vi "FPGA_v1.vi"() -> ()   [LabVIEW 2017]
panel:
  out "T":sgl
  in  "h":sgl format="%#_13g"
  out "norm(V)":sgl
  out "AoA_Yaw":sgl
  out "AoA_Pitch":sgl
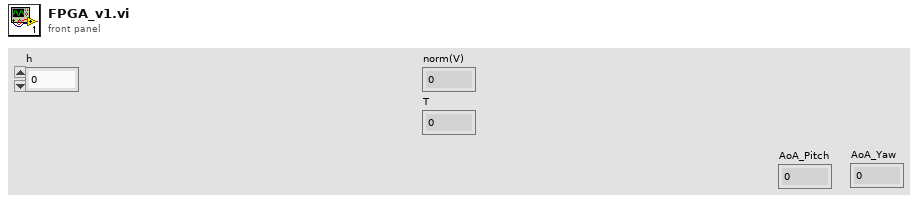
[diagram p1: front panel]
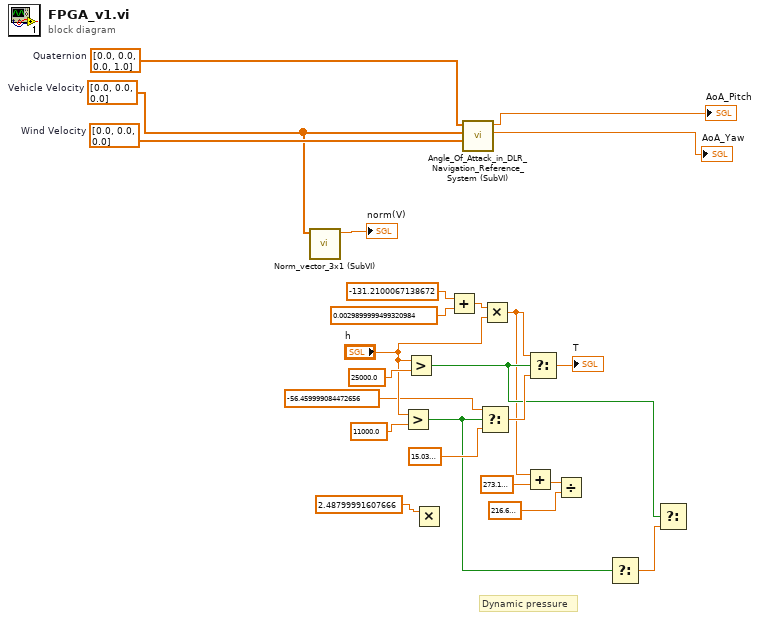
[diagram p0: block diagram]
diagram:
  w23 = sgl[] [0.0, 0.0, 0.0]  # Wind Velocity
  w20 = sgl[] [0.0, 0.0, 0.0]  # Vehicle Velocity
  w24 = sgl[] [0.0, 0.0, 0.0, 1.0]  # Quaternion
  # "Dynamic pressure"
  n1 = call "Norm_vector_3x1 (SubVI).vi"("Vector"=w20) -> ("Norm"=→"norm(V)":sgl)  [unwired: 10 in]
  n2 = Greater?(x="h", y=sgl 11000.0) -> (0:w6:bool)
  n3 = Greater?(x="h", y=sgl 25000.0) -> (0:w7:bool)
  n4 = Multiply(x=sgl 2.488 ("t")) -> ()  [unwired: 1 in, 1 out]
  n5 = Add(x=sgl -131.21, y=sgl 0.00299) -> (x+y=w17:sgl)
  n6 = call "Angle_Of_Attack_in_DLR_Navigation_Reference_System (SubVI).vi"("Wind Velocity"=w23, "Vehicle Velocity"=w20, "Quaternion"=w24) -> ("AoA Yaw"=→"AoA_Yaw":sgl, "AoA Pitch"=→"AoA_Pitch":sgl)  [unwired: 7 in]
  n7 = Select(t=sgl -56.46, s=w6, f=sgl 15.04) -> (s? t:f=w11:sgl)
  n8 = Multiply(x=w17, y="h") -> (x*y=w4:sgl)
  n9 = Add(x=w4, y=sgl 273.1) -> (x+y=w2:sgl)
  n10 = Select(t=w4, s=w7, f=w11) -> (s? t:f=→"T":sgl)
  n11 = Divide(x=w2, y=sgl 216.6) -> ()  [unwired: 1 out]
  n12 = Select(s=w6) -> (s? t:f=w9:dbl)  [unwired: 2 in]
  n13 = Select(s=w7, f=w9) -> ()  [unwired: 1 in, 1 out]
